vi "VRM Axis to Axis Array.vi"(1 "Axis":T1) -> (0 "Axis Array":T2[](array[typedef]))   [LabVIEW 2019, in "Instrument.OxfordVRM.lvclass"]
uses:
  Instrument.OxfordVRM.lvclass
  <userlib>/LevyLab/Instrument Framework/Instrument Types/Cryostat/Typedefs/Magnet Axis--Enum.ctl
  Typedefs/VRM Magnet Axis--Enum.ctl
  <userlib>/LevyLab/Instrument Framework/Instrument Types/Cryostat/Instrument.Cryostat.lvclass
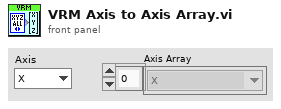
[diagram p1: front panel]
types:
  T1 = typedef "Instrument.OxfordVRM.lvclass/VRM Magnet Axis--Enum.ctl" = enum16{"X", "Y", "Z", "ALL"}
  T2 = typedef "Instrument.Cryostat.lvclass/Magnet Axis--Enum.ctl" = enum16{"X", "Y", "Z"}
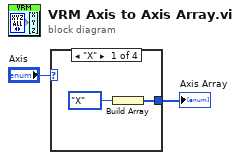
[diagram p0: block diagram]
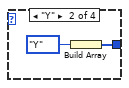
[diagram p2: hidden frame]
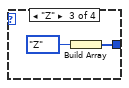
[diagram p3: hidden frame]
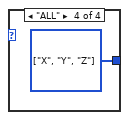
[diagram p4: hidden frame]
diagram:
  n1 = case shown="\"X\"" "Axis" {
    tunnel: [w3 w5 w7 w9] -> w2
    frame "X" {
      n2 = Build Array(Magnet_Axis--Enum."X" ("Axis")) -> (w3:T2[])
    }
    frame "Y" {
      n3 = Build Array(Magnet_Axis--Enum."Y" ("Axis")) -> (w5:T2[])
    }
    frame "Z" {
      n4 = Build Array(Magnet_Axis--Enum."Z" ("Axis")) -> (w7:T2[])
    }
    frame "ALL" {
      w9 = T2[] [enum."X", enum."Y", enum."Z"] items=["X", "Y", "Z"] ("Array")
    }
  }
  "Axis Array" <- w2
